vi "CHECK Color V3.vi"(8 "error in (no error)":errorcluster, 11 "refnum name":string) -> (0 "error out":errorcluster, 1 "Proximity":u16, 2 "Matched Color Name":string, 3 "ColorSensorDevRef out":T1={"I2CDevRef"={"DevStatus"={"status"=FALSE, "code"=0, "source"=""}, "Device Address"=0, "Handle"=0, "I2C Bus"=enum."Invalid"}} {"I2CDevRef"."Device Address" format="%.0x"}, 4 "Confidence":dbl)   [LabVIEW 2020]
uses:
  <vilib>/Rock Robotics/WPI/ThirdParty/REV Robotics/REVLib/Typedef/Color Sensor V3 DevRef.ctl
  <vilib>/Rock Robotics/WPI/I2C/WPI_I2CDevRef.ctl
  <vilib>/Rock Robotics/SystemInterfaces/i2clib/i2c_bus.ctl
  <vilib>/Rock Robotics/Network Tables/NT Write String.vi
  <vilib>/Rock Robotics/Network Tables/NT Write Number.vi
  <vilib>/Rock Robotics/Network Tables/NT Write Numeric Array.vi
  <vilib>/Rock Robotics/Network Tables/NT Read String.vi
  <vilib>/Rock Robotics/Network Tables/NT Write Boolean.vi
panel:
  out "Matched Color":cluster{"R":dbl, "G":dbl, "B":dbl}
  out "Normalized Color":cluster{"R":dbl, "G":dbl, "B":dbl}
  out "Color":u32(colorbox)
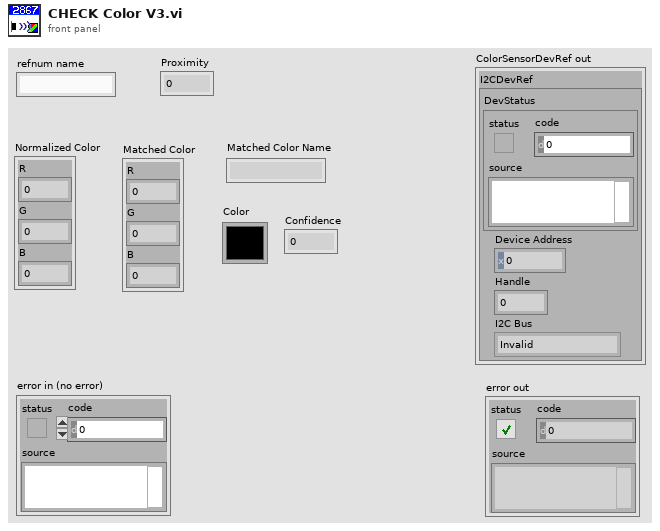
[diagram p1: front panel]
types:
  T1 = typedef "Color Sensor V3 DevRef.ctl" = cluster{"I2CDevRef":T2}
  T2 = typedef "WPI_I2CDevRef.ctl" = cluster{"DevStatus":errorcluster, "Device Address":u8, "Handle":i32, "I2C Bus":T3}
  T3 = typedef "i2c_bus.ctl" = enum16{"I2C On-Board", "I2C MXP", "Invalid"}
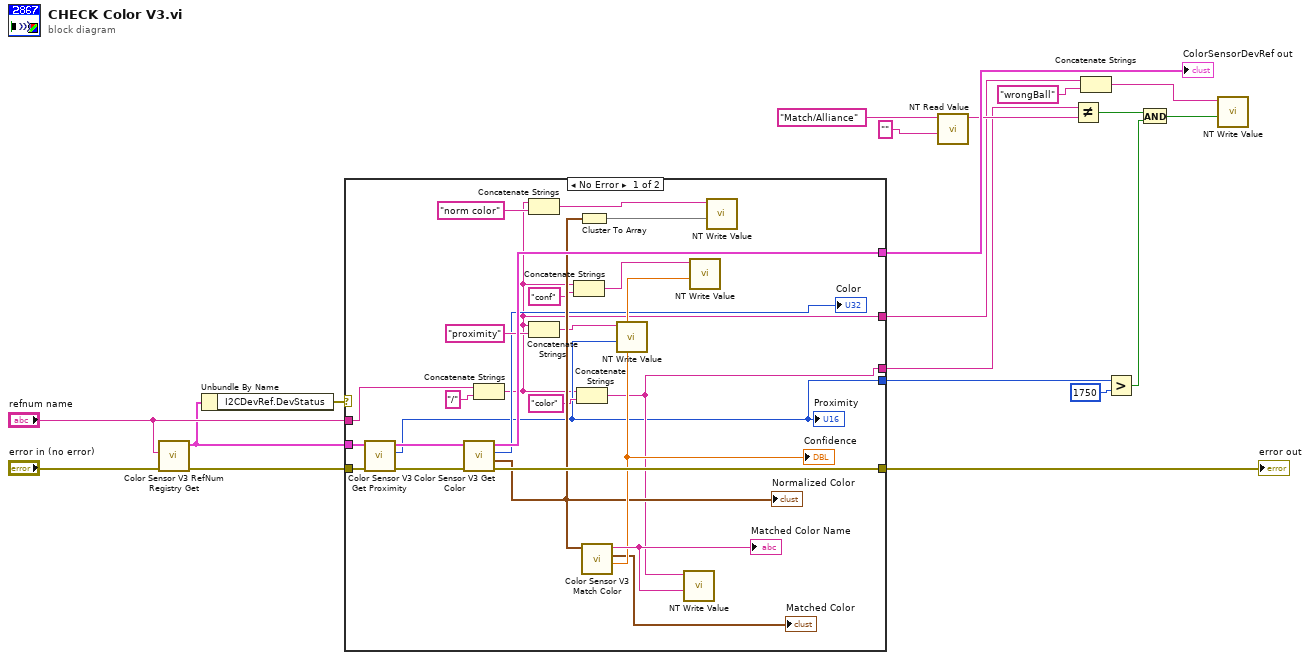
[diagram p0: block diagram]
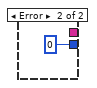
[diagram p2: hidden frame]
diagram:
  n1 = call <vilib>:"Color Sensor V3 RefNum Registry Get.vi"("error in (no error)"="error in (no error)", "refnum name"="refnum name") -> ("error out"=w15:errorcluster, "ColorSensorDevRef"=w14:T1)  [unwired: 8 in]
  n2 = Unbundle By Name(w14) -> ("I2CDevRef.DevStatus"=w13:errorcluster)
  n3 = case shown="No Error" w13 {
    tunnel: "refnum name" -> [w43 _]
    tunnel: [w42 _] -> w18
    tunnel: [w41 _] -> w17
    tunnel: w15 -> [w40 _]
    tunnel: w14 -> [w39 _]
    tunnel: [w22 _] -> w9
    tunnel: [w21 u16 0 ("Proximity")] -> w8
    tunnel: [w20 _] -> w1
    frame No Error {
      n4 = call <vilib>:"Color Sensor V3 Get Proximity.vi"("error in (no error)"=w40, "ColorSensorDevRef"=w39) -> ("error out"=w38:errorcluster, "Proximity"=w21:u16, "ColorSensorDevRef out"=w37:T1)  [unwired: 7 in]
      "Proximity" <- w21
      n5 = call <vilib>:"Color Sensor V3 Get Color.vi"("error in (no error)"=w38, "ColorSensorDevRef"=w37) -> ("error out"=w42:errorcluster, "Normalized Color"=w34:cluster{"R":dbl, "G":dbl, "B":dbl}, "Color"=→"Color":u32, "ColorSensorDevRef out"=w41:T1)  [unwired: 6 in]
      "Normalized Color" <- w34
      n6 = Concatenate Strings(w43, "/" ("string")) -> (w20:string)
      n7 = Concatenate Strings(w20, "norm color" ("string")) -> (w30:string)
      n8 = Concatenate Strings(w20, "proximity" ("string")) -> (w31:string)
      n9 = Concatenate Strings(w20, "conf" ("string")) -> (w29:string)
      n10 = Concatenate Strings(w20, "color" ("string")) -> (w22:string)
      n11 = Cluster To Array(cluster=w34) -> (array=w33:dbl[])
      n12 = call <vilib>:"Color Sensor V3 Match Color.vi"("Measured Color"=w34) -> ("Confidence"=w35:dbl, "Matched Color"=→"Matched Color":cluster{"R":dbl, "G":dbl, "B":dbl}, "Matched Color Name"=w36:string)  [unwired: 8 in]
      "Confidence" <- w35
      "Matched Color Name" <- w36
      n13 = call-poly <vilib>:"NT Write Value.vi"("Numeric"=w21, "Name"=w31) -> ()  [unwired: 9 in, 1 out]
      n14 = call-poly <vilib>:"NT Write Value.vi"("String"=w36, "Name"=w22) -> ()  [unwired: 9 in, 1 out]
      n15 = call-poly <vilib>:"NT Write Value.vi"("Numeric"=w35, "Name"=w29) -> ()  [unwired: 9 in, 1 out]
      n16 = call-poly <vilib>:"NT Write Value.vi"("Numeric Array"=w33, "Name"=w30) -> ()  [unwired: 9 in, 1 out]
    }
    frame Error {
    }
  }
  "error out" <- w18
  "ColorSensorDevRef out" <- w17
  n17 = call-poly <vilib>:"NT Read Value.vi"("Default Value"="", "Name"="Match/Alliance") -> ("String"=w10:string)  [unwired: 8 in, 1 out]
  n18 = Not Equal?(x=w9, y=w10) -> (x != y?=w5:bool)
  n19 = Concatenate Strings(w1, "wrongBall" ("Name")) -> (w2:string)
  n20 = Greater?(x=w8, y=u16 1750) -> (0:w6:bool)
  n21 = And(x=w5, y=w6) -> (x .and. y?=w4:bool)
  n22 = call-poly <vilib>:"NT Write Value.vi"("Boolean"=w4, "Name"=w2) -> ()  [unwired: 9 in, 1 out]
